vi "Write_a_Crypted_File.vi"(7 "name of Folder":string, 8 "error in (no error)":errorcluster, 9 "name of file":string, 10 "Encrypted text":string, 11 "object in":refnum<class "Crypter.lvclass">) -> (0 "error out":errorcluster, 3 "object out":refnum<class "Crypter.lvclass">)   [LabVIEW 2016, in "Crypter.lvclass"]
uses:
  Crypter.lvclass
  Crypter.lvclass/Crypter.ctl
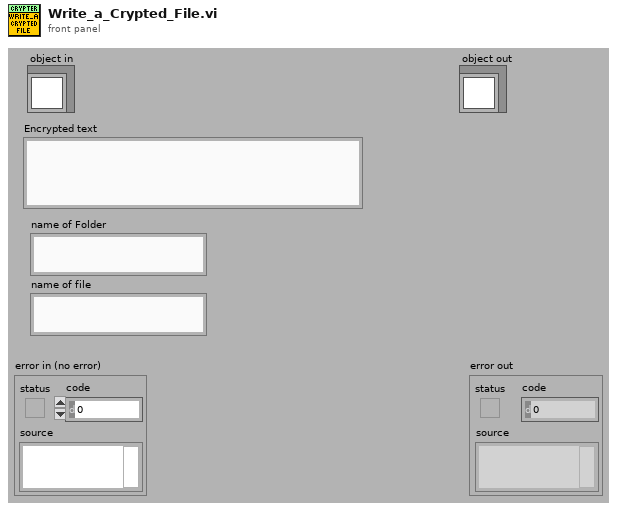
[diagram p1: front panel]
types:
  T1 = enum16{"open", "replace", "create", "open or create", "replace or create", "replace or create with confirmation"}
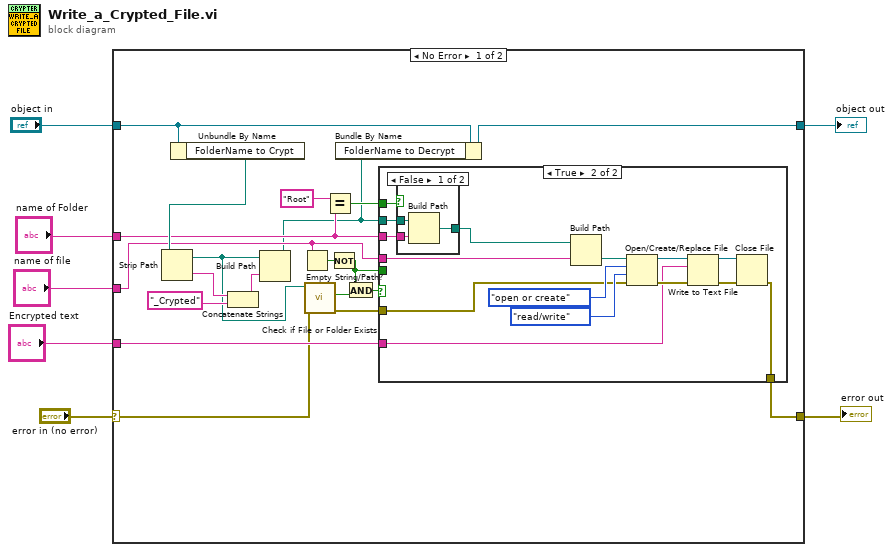
[diagram p0: block diagram]
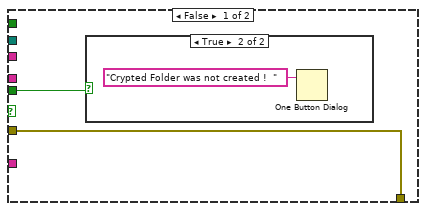
[diagram p2: hidden frame]
diagram:
  n1 = case shown="No Error" "error in (no error)" {
    selector: "error in (no error)" -> [w19 w51]
    tunnel: [w18 w51] -> w6
    tunnel: [w9 w50] -> w4
    tunnel: "object in" -> [w27 w50]
    tunnel: "name of Folder" -> [w17 _]
    tunnel: "Encrypted text" -> [w26 _]
    tunnel: "name of file" -> [w13 _]
    frame No Error {
      n2 = Unbundle By Name(w27) -> ("FolderName to Crypt"=w22:path)
      n3 = Strip Path(path=w22) -> (stripped path=w21:path, name=w24:string)
      n4 = Concatenate Strings(w24, "_Crypted") -> (w23:string)
      n5 = Build Path(base path=w21, name or relative path=w23) -> (appended path=w8:path)
      n6 = Empty String/Path?(string/path=w13) -> (empty?=w12:bool)
      n7 = call <vilib>:"Check if File or Folder Exists.vi"("error in (no error)"=w19, "path"=w21) -> ("error out"=w20:errorcluster, "file or folder exists?"=w14:bool)  [unwired: 7 in, 1 out]
      n8 = Equal?(x="Root", y=w17) -> (x = y?=w15:bool)
      n9 = Not(x=w12) -> (.not. x?=w10:bool)
      n10 = Bundle By Name(cluster=w27, "FolderName to Decrypt"=w8) -> (w9:refnum<class "Crypter.lvclass">)
      n11 = And(x=w10, y=w14) -> (x .and. y?=w11:bool)
      n12 = case shown="True" w11 {
        tunnel: w17 -> [_ w39]
        tunnel: w26 -> [_ w38]
        tunnel: w8 -> [_ w37]
        tunnel: w20 -> [w29 w31]
        tunnel: [w29 w36] -> w18
        tunnel: w13 -> [_ w34]
        tunnel: w15 -> [_ w33]
        tunnel: w10 -> [w28 _]
        frame False {
          n13 = case shown="True" w28 {
            frame False {
            }
            frame True {
              n14 = One Button Dialog(message="Crypted Folder was not created !  ") -> ()  [unwired: 1 in, 1 out]
            }
          }
        }
        frame True {
          n15 = case shown="False" w33 {
            tunnel: w39 -> [w48 _]
            tunnel: w37 -> [w47 w49]
            tunnel: [w46 w49] -> w35
            frame False {
              n16 = Build Path(base path=w47, name or relative path=w48) -> (appended path=w46:path)
            }
            frame True {
            }
          }
          n17 = Build Path(base path=w35, name or relative path=w34) -> (appended path=w32:path)
          n18 = Open/Create/Replace File(file path (use dialog)=w32, error in=w31, operation (0:open)=T1."open or create", access (0:read/write)=enum16{"read/write", "read-only", "write-only"}."read/write") -> (refnum out=w43:refnum<file>, error out=w42:errorcluster)  [unwired: 2 in, 1 out]
          n19 = Write to Text File(file (use dialog)=w43, text=w38, error in=w42) -> (refnum out=w40:refnum<file>, error out=w41:errorcluster)  [unwired: 1 in, 1 out]
          n20 = Close File(refnum=w40, error in=w41) -> (error out=w36:errorcluster)  [unwired: 1 out]
        }
      }
    }
    frame Error {
    }
  }
  "error out" <- w6
  "object out" <- w4
